vi "Measure DC Volts.vi"(10 "measurementservice_DMMConfigRequest_Data":T1, 11 "IVI Refnum in":refnum<k15>="DMM" caption="Device Name") -> (0 "error out":errorcluster, 3 "Measurement (Volts)":dbl format="%_7p")   [LabVIEW 2019, in "HVC2.lvlib" / "HVC2.lvclass"]
uses:
  HVC2 Class/HVC2.lvclass
  HVC2 Class/RPC Messages/measurementservice_DMMConfigRequest/measurementservice_DMMConfigRequest_Data.ctl
  <instrlib>/niDMM/nidmm.llb/niDMM Configure Measurement Digits.vi
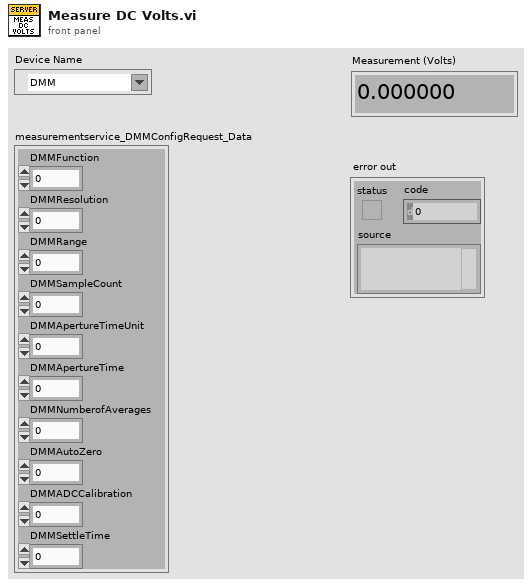
[diagram p1: front panel]
types:
  T1 = typedef "HVC2.lvlib/HVC2.lvclass/measurementservice_DMMConfigRequest_Data.ctl" = cluster{"DMMFunction":i32, "DMMResolution":sgl, "DMMRange":sgl, "DMMSampleCount":i32, "DMMApertureTimeUnit":i32, "DMMApertureTime":sgl, "DMMNumberofAverages":i32, "DMMAutoZero":i32, "DMMADCCalibration":i32, "DMMSettleTime":sgl}
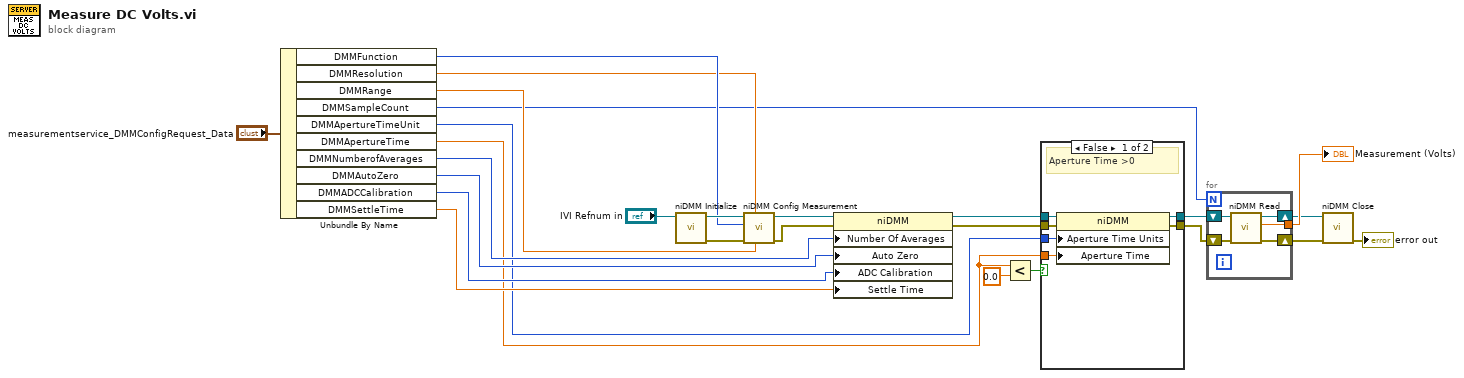
[diagram p0: block diagram]
diagram:
  n1 = Unbundle By Name("measurementservice_DMMConfigRequest_Data") -> ("DMMFunction"=w18:i32, "DMMResolution"=w17:sgl, "DMMRange"=w16:sgl, "DMMSampleCount"=w15:i32, "DMMApertureTimeUnit"=w2:i32, "DMMApertureTime"=w1:sgl, "DMMNumberofAverages"=w12:i32, "DMMAutoZero"=w11:i32, "DMMADCCalibration"=w10:i32, "DMMSettleTime"=w9:sgl)
  n2 = call <instrlib>:"niDMM Initialize.vi"("Instrument Descriptor"="IVI Refnum in") -> ("error out"=w24:errorcluster, "instrument handle out"=w25:refnum<k15>)  [unwired: 9 in]
  n3 = call-poly <instrlib>:"niDMM Config Measurement.vi"("Range"=w16, "Resolution in Digits"=w17, "error in (no error)"=w24, "Function"=w18, "instrument handle"=w25) -> ("error out"=w13:errorcluster, "instrument handle out"=w14:refnum<k15>)  [unwired: 5 in]
  n4 = property class="niDMM"(reference=w14, error in=w13, "Number Of Averages"=w12, "Auto Zero"=w11, "ADC Calibration"=w10, "Settle Time"=w9) -> (reference out=w8:refnum<k15>, error out=w7:errorcluster)
  n5 = Less?(x=w1, y=0.0 ("Configuration:Advanced:Aperture Time")) -> (x < y?=w3:bool)
  n6 = case shown="False" w3 {
    tunnel: w8 -> [w32 w34]
    tunnel: w7 -> [w31 w33]
    tunnel: [w30 w34] -> w6
    tunnel: [w29 w33] -> w5
    tunnel: w2 -> [w28 _]
    tunnel: w1 -> [w27 _]
    frame False {
      # "Aperture Time >0"
      n7 = property class="niDMM"(reference=w32, error in=w31, "Aperture Time Units"=w28, "Aperture Time"=w27) -> (reference out=w30:refnum<k15>, error out=w29:errorcluster)
    }
    frame True {
      # "Aperture Time <0"
    }
  }
  n8 = for {
    N: w15 -> [_]
    tunnel: [w39] -> w22
    shift-right: [w37] -> w20
    shift-left: w5 -> [w36]
    shift-right: [w38] -> w21
    shift-left: w6 -> [w35]
    n9 = call <instrlib>:"niDMM Read.vi"("error in (no error)"=w36, "instrument handle"=w35) -> ("error out"=w37:errorcluster, "Measurement"=w39:dbl, "instrument handle out"=w38:refnum<k15>)  [unwired: 7 in]
  }
  "Measurement (Volts)" <- w22
  n10 = call <instrlib>:"niDMM Close.vi"("error in (no error)"=w20, "instrument handle"=w21) -> ("error out"=→"error out":errorcluster)  [unwired: 9 in]
